vi "Read sPanel.vi"(8 "error in (no error)":errorcluster, 11 "GUI Facade in":refnum<class "GUI Facade.lvclass">) -> (0 "error out":errorcluster, 2 "sPanel":refnum<vi>, 3 "GUI Facade out":refnum<class "GUI Facade.lvclass">)   [LabVIEW 2018, in "GUI Facade.lvclass"]
uses:
  GUI Facade.lvclass
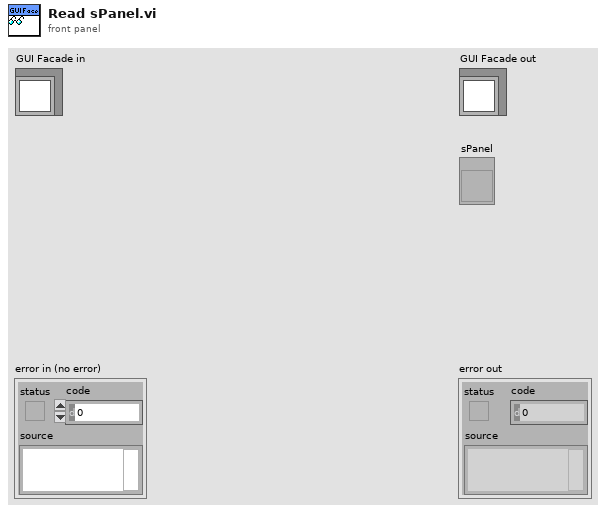
[diagram p1: front panel]
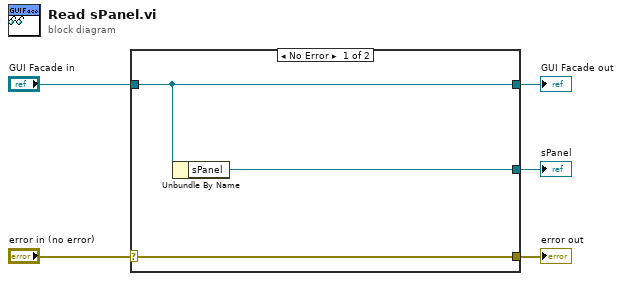
[diagram p0: block diagram]
diagram:
  n1 = case shown="No Error" "error in (no error)" {
    selector: "error in (no error)" -> [w8 w9]
    tunnel: [w8 w9] -> w4
    tunnel: [w7 w10] -> w2
    tunnel: "GUI Facade in" -> [w7 w10]
    tunnel: [w6 _] -> w1
    frame No Error {
      n2 = Unbundle By Name(w7) -> ("sPanel"=w6:refnum<vi>)
    }
    frame Error {
    }
  }
  "error out" <- w4
  "GUI Facade out" <- w2
  "sPanel" <- w1
